vi "CheckCollision.vi"(8 "error in":errorcluster, 10 "sprite in":refnum<class "Sprite.lvclass">, 11 "class data in":refnum<class "Paddle.lvclass">) -> (0 "error out":errorcluster, 1 "collisionInfo out":cluster{"collision":bool, "fatal":bool}, 2 "sprite out":refnum<class "Sprite.lvclass">, 3 "class data out":refnum<class "Paddle.lvclass">)   [LabVIEW 2010, in "Labricks.lvlib" / "Paddle.lvclass"]
uses:
  Paddle.lvclass
  RenderBase/Sprite_class/Sprite.lvclass
  RenderBase/SceneObject_class/CollisionAction.ctl
  RenderBase/SceneRoot_class/SceneRoot.lvclass
  RenderBase/SceneObject_class/properties/SceneRoot/GetSceneRoot.vi
  RenderBase/SceneObject_class/properties/Position/GetPosition.vi
  RenderBase/SceneObject_class/SceneObject.lvclass
  <vilib>/picture/3D Picture Control/NI_3D Picture Control.lvlib
  Game_class/Game.lvclass
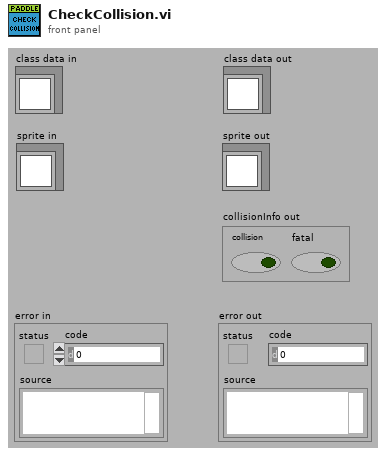
[diagram p1: front panel]
types:
  T1 = typedef "RenderBase.lvlib/SceneObject.lvclass/CollisionAction.ctl" = enum16{"None", "BounceX", "BounceY", "BounceXY"}
  T2 = typedef "LV3DPointTypeDef.ctl" = cluster{"X":sgl, "Y":sgl, "Z":sgl}
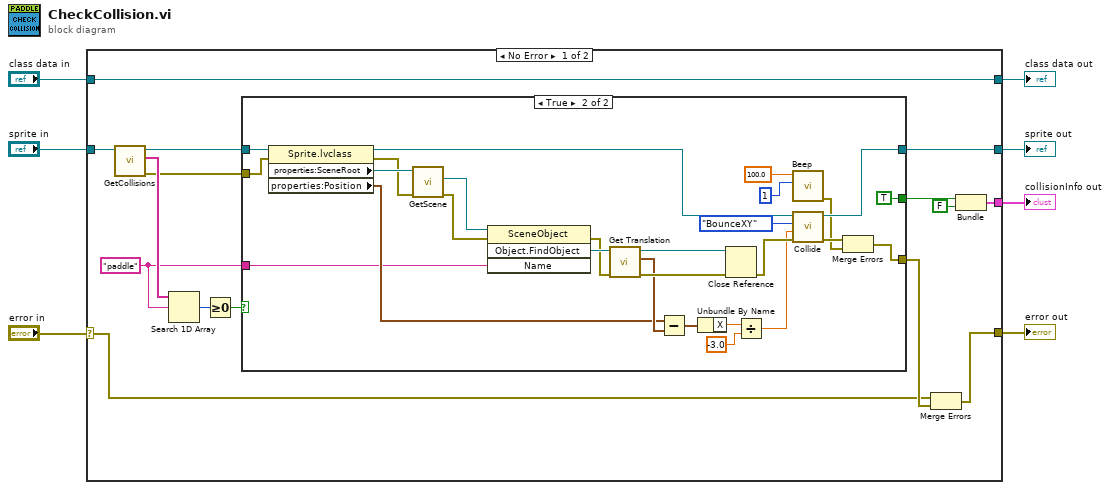
[diagram p0: block diagram]
diagram:
  n1 = case shown="No Error" "error in" {
    selector: "error in" -> [w17 w54]
    tunnel: [w18 w54] -> w7
    tunnel: "sprite in" -> [w12 w52]
    tunnel: [w21 w53] -> w5
    tunnel: "class data in" -> [w21 w53]
    tunnel: [w19 w52] -> w2
    tunnel: [w16 _] -> w1
    frame No Error {
      w8 = "paddle" ("search string")
      n2 = call-dynamic "GetCollisions.vi"("sprite in"=w12) -> ("error out"=w9:errorcluster, "collisions out"=w14:string[], "sprite out"=w11:refnum<class "Sprite.lvclass">)  [unwired: 8 in]
      n3 = Search 1D Array(1D array=w14, element=w8) -> (index of element=w13:i32)  [unwired: 1 in]
      n4 = Greater Or Equal To 0?(x=w13) -> (x >= 0?=w10:bool)
      n5 = case shown="True" w10 {
        tunnel: [w23 w39] -> w22
        tunnel: [_ TRUE] -> w20
        tunnel: w11 -> [w24 w35]
        tunnel: [w24 w50] -> w19
        tunnel: w9 -> [w23 w33]
        tunnel: w8 -> [_ w31]
        frame False {
        }
        frame True {
          n6 = property class="Sprite.lvclass"(reference=w35, error in=w33) -> (reference out=w34:refnum<class "Sprite.lvclass">, error out=w27:errorcluster, "properties:SceneRoot"=w28:refnum<class "SceneRoot.lvclass">, "properties:Position"=w32:T2)
          n7 = call "GetScene.vi"("error in (no error)"=w27, "reference in"=w28) -> ("error out"=w25:errorcluster, "Scene"=w26:refnum<vi>)  [unwired: 7 in, 1 out]
          n8 = invoke class="SceneObject" method="Object.FindObject"(reference=w26, error in=w25, "Name"=w31) -> (error out=w29:errorcluster, "FindObject"=w30:refnum<vi>)  [unwired: 1 in, 2 out]
          n9 = call <vilib>:"Get Translation.vi"("error in (no error)"=w29, "Scene Object"=w30) -> ("error out"=w46:errorcluster, "Transformation:Get Translation"=w43:cluster{"X":sgl, "Y":sgl, "Z":sgl}, "Scene Object"=w45:refnum<vi>)  [unwired: 7 in]
          n10 = Subtract(x=w32, y=w43) -> (x-y=w44:T2)
          n11 = Unbundle By Name(w44) -> ("X"=w42:sgl)
          n12 = Close Reference(reference=w45, error in (no error)=w46) -> (error out=w47:errorcluster)
          n13 = Divide(x=w42, y=sgl -3.0) -> (x/y=w40:sgl)
          n14 = call "Beep.vi"("numChunks in"=1 ("#s"), "frequency in"=100.0 ("frequency")) -> ("error out"=w36:errorcluster)  [unwired: 9 in]
          n15 = call-dynamic "Collide.vi"("error in (no error)"=w47, "angleCorrection in"=w40, "action in"=CollisionAction."BounceXY", "class data in"=w34) -> ("error out"=w49:errorcluster, "class data out"=w50:refnum<class "Sprite.lvclass">)  [unwired: 6 in]
          n16 = Merge Errors(w49, w36) -> (w39:errorcluster)
        }
      }
      n17 = Merge Errors(w17, w22) -> (w18:errorcluster)
      n18 = Bundle(w20, FALSE) -> (w16:cluster{bool, bool})  [unwired: 1 in]
    }
    frame Error {
    }
  }
  "error out" <- w7
  "class data out" <- w5
  "sprite out" <- w2
  "collisionInfo out" <- w1
